vi "FTP Send Whole Directory.vi"(10 "Local Folder of Autonomous Plays":path, 11 "host":string="10.26.14.21") -> (0 "error out":errorcluster)   [LabVIEW 2014]
uses:
  <vilib>/FTP/NI_FTP.lvlib
panel:
  in  "Target Remote directory path":string="/Autonomous-Plays"
  in  "password":string
  in  "user":string="anonymous"
  out "file errors":errorcluster[](array[cluster])
  out "Converted DIR Specifications":T1(array[cluster])
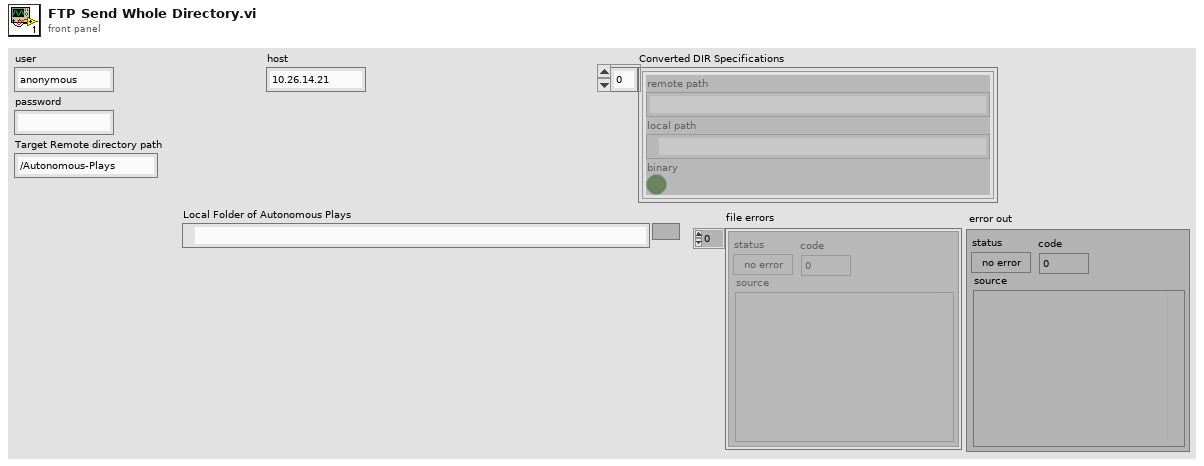
[diagram p1: front panel]
types:
  T1 = cluster{"remote path":string, "local path":path, "binary":bool}[]
  T2 = cluster{"remote path":string, "local path":path, "binary":bool}
  T3 = typedef "NI_FTP.lvlib/FTP Session.ctl" = refnum<k5>
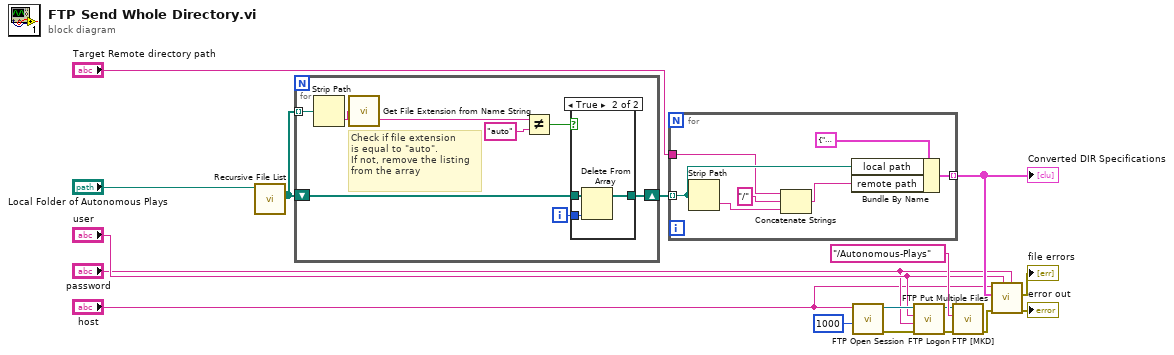
[diagram p0: block diagram]
diagram:
  n1 = call <vilib>:"Recursive File List.vi"("Folder Path"="Local Folder of Autonomous Plays") -> ("All Files in Dir"=w17:path[])  [unwired: 6 in, 4 out]
  n2 = for {
    tunnel: w17 -> [w20] mode=indexing
    shift-right: [w18] -> w15
    shift-left: w17 -> [w24]
    i -> [w22]
    # "Check if file extension\nis equal to \"auto\".\nIf not, remove the listing\nfrom the array"
    n3 = Strip Path(path=w20) -> (name=w19:string)  [unwired: 1 out]
    n4 = call "Get File Extension from Name String.vi"("File Name String"=w19) -> ("lowercase file extension"=w21:string)  [unwired: 1 out]
    n5 = Not Equal?(x=w21, y="auto") -> (x != y?=w23:bool)
    n6 = case shown="True" w23 {
      tunnel: w24 -> [w26 w28]
      tunnel: w22 -> [_ w29]
      tunnel: [w26 w27] -> w18
      frame False {
      }
      frame True {
        n7 = Delete From Array(array=w28, index=w29) -> (array with subset deleted=w27:path[])  [unwired: 1 in, 1 out]
      }
    }
  }
  n8 = for {
    tunnel: w15 -> [w35] mode=indexing
    tunnel: "Target Remote directory path" -> [w34]
    tunnel: [w30] -> w11 mode=indexing
    n9 = Strip Path(path=w35) -> (name=w32:string)  [unwired: 1 out]
    n10 = Concatenate Strings(w34, "/" ("string"), w32) -> (w31:string)
    n11 = Bundle By Name(cluster=T2 {"remote path"="", "local path"=path "", "binary"=FALSE} ("transfer spec"), "local path"=w35, "remote path"=w31) -> (w30:T2)
  }
  "Converted DIR Specifications" <- w11
  n12 = call <vilib>:"FTP Open Session.vi"("timeout ms (60000)"=1000, "address"="host") -> ("error out"=w8:errorcluster, "ftp session"=w9:T3)  [unwired: 6 in, 2 out]
  n13 = call <vilib>:"FTP Logon.vi"("error in (no error)"=w8, "password"="password", "user"="user", "ftp session"=w9) -> ("error out"=w6:errorcluster, "ftp session out"=w7:T3)  [unwired: 4 in, 2 out]
  n14 = call <vilib>:"FTP [MKD].vi"("error in (no error)"=w6, "directory path"="/Autonomous-Plays", "ftp session"=w7) -> ("error out"=w2:errorcluster)  [unwired: 5 in, 3 out]
  n15 = call <vilib>:"FTP Put Multiple Files.vi"("password"="password", "user"="user", "error in (no error)"=w2, "file specifications"=w11, "host"="host") -> ("error out"=→"error out":errorcluster, "file errors"=→"file errors":errorcluster[])  [unwired: 5 in]
